vi "test Write rtlinux.vi"() -> ()   [LabVIEW 2026]
uses:
  source/PCANBasic.lvlib
  source/PCAN Message types.ctl
  source/PCAN Message.ctl
  source/TPCANHandle.ctl
  source/PCAN Baud.ctl
panel:
  out "error out":errorcluster
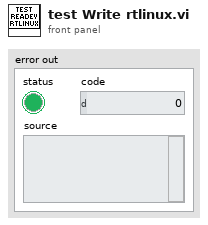
[diagram p1: front panel]
types:
  T1 = typedef "PCANBasic.lvlib/PCAN Baud.ctl" = u16
  T2 = typedef "PCANBasic.lvlib/TPCANHandle.ctl" = u16
  T3 = typedef "PCANBasic.lvlib/PCAN Message.ctl" = cluster{"ID":u32, "MSGTYPE":T4, "LEN":u8, "DATA":cluster{"0":u8, "1":u8, "2":u8, "3":u8, "4":u8, "5":u8, "6":u8, "7":u8}}
  T4 = typedef "PCANBasic.lvlib/PCAN Message types.ctl" = u8
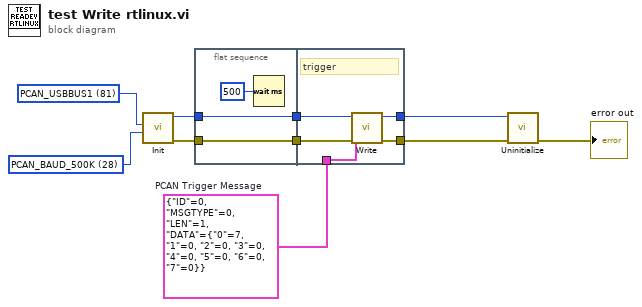
[diagram p0: block diagram]
diagram:
  w5 = T1 28 items=["PCAN_BAUD_1M"=20, "PCAN_BAUD_800K"=22, "PCAN_BAUD_500K"=28, "PCAN_BAUD_250K"=284, "PCAN_BAUD_125K"=796, "PCAN_BAUD_100K"=17199, "PCAN_BAUD_95K"=49998, "PCAN_BAUD_83K"=34091, "PCAN_BAUD_50K"=18223, "PCAN_BAUD_47K"=5140, "PCAN_BAUD_33K"=35631, "PCAN_BAUD_20K"=21295, "PCAN_BAUD_10K"=26415, "PCAN_BAUD_5K"=32639] ("Baudrate")
  w6 = T2 81 items=["PCAN_NONEBUS"=0, "PCAN_USBBUS1"=81, "PCAN_USBBUS2"=82, "PCAN_USBBUS3"=83, "PCAN_USBBUS4"=84, "PCAN_USBBUS5"=85, "PCAN_USBBUS6"=86, "PCAN_USBBUS7"=87, "PCAN_USBBUS8"=88, "PCAN_USBBUS9"=1289, "PCAN_USBBUS10"=1290, "PCAN_USBBUS11"=1291, "PCAN_USBBUS12"=1292, "PCAN_USBBUS13"=1293, "PCAN_USBBUS14"=1294, "PCAN_USBBUS15"=1295, "PCAN_USBBUS16"=1296] ("Channel")
  w8 = T3 {"ID"=0, "MSGTYPE"=0, "LEN"=1, "DATA"={"0"=7, "1"=0, "2"=0, "3"=0, "4"=0, "5"=0, "6"=0, "7"=0}}  # PCAN Trigger Message
  n1 = call "Init.vi"("Baudrate"=w5, "Channel"=w6) -> ("error out"=w3:errorcluster, "TPCANHandle out"=w2:T2)  [unwired: 7 in, 1 out]
  n2 = flat-sequence {
    tunnel: w2 -> [w12]
    tunnel: [w12] -> w10
    tunnel: w3 -> [w11]
    tunnel: [w11] -> w9
    tunnel: w10 -> [w18]
    tunnel: w9 -> [w17]
    tunnel: [w16] -> w7
    tunnel: w8 -> [w15]
    tunnel: [w14] -> w1
    frame #0 {
      n3 = Wait (ms)(milliseconds to wait=u32 500) -> ()  [unwired: 1 out]
    }
    frame #1 {
      # "trigger"
      n4 = call "Write.vi"("error in"=w17, "PCAN Message"=w15, "TPCANHandle in"=w18) -> ("error out"=w16:errorcluster, "TPCANHandle out"=w14:T2)  [unwired: 6 in, 1 out]
    }
  }
  n5 = call "Uninitialize.vi"("error in"=w7, "TPCANHandle in"=w1) -> ("error out"=→"error out":errorcluster)  [unwired: 8 in, 1 out]
